vi "CM_DetectPulses.vi"(8 "Error In":errorcluster, 11 "Data":dbl[][](array[numeric])) -> (0 "Error out":errorcluster)   [LabVIEW 2016]
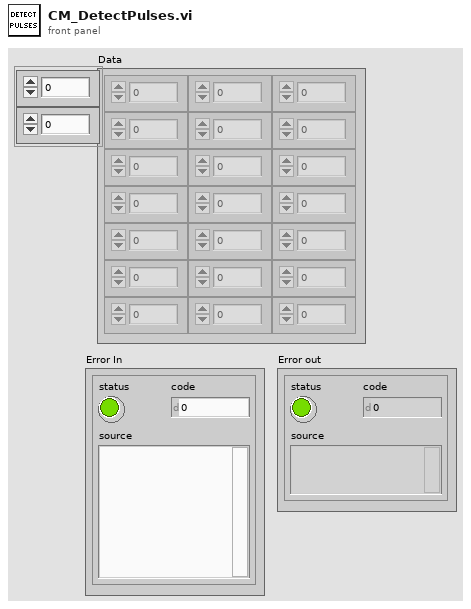
[diagram p1: front panel]
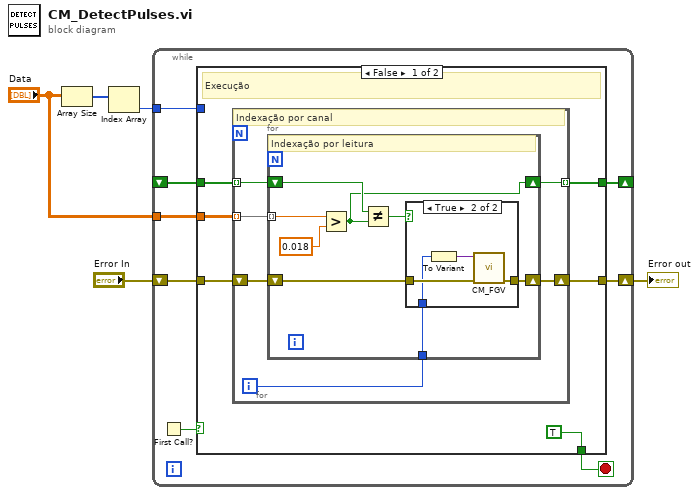
[diagram p0: block diagram]
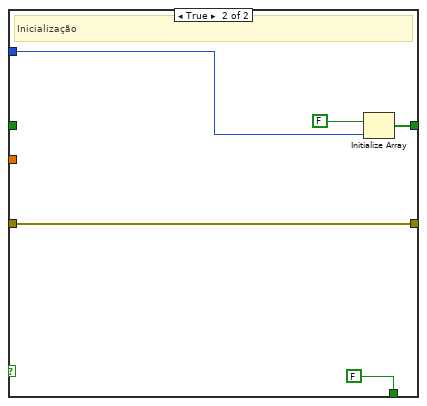
[diagram p3: hidden frame]
diagram:
  n1 = Array Size(array="Data") -> (size(s)=w5:i32[])
  n2 = Index Array(array=w5) -> (element=w4:i32)  [unwired: 1 in]
  n3 = while {
    tunnel: w4 -> [w12]
    shift-right: [w11] -> _
    shift-left: _ -> [w10]
    tunnel: "Data" -> [w9]
    shift-right: [w8] -> w1
    shift-left: "Error In" -> [w7]
    stop <- w13 stop-if-true
    n4 = First Call?() -> (First Call?: T/F=w6:bool)
    n5 = case shown="False" w6 {
      tunnel: [TRUE FALSE] -> w13
      tunnel: w12 -> [_ w42]
      tunnel: [w14 w40] -> w11
      tunnel: w10 -> [w18 _]
      tunnel: w9 -> [w17 _]
      tunnel: [w16 w39] -> w8
      tunnel: w7 -> [w15 w39]
      frame False {
        # "Execução"
        n6 = for {
          tunnel: w18 -> [w25] mode=indexing
          tunnel: w17 -> [w24] mode=indexing
          shift-right: [w23] -> w16
          shift-left: w15 -> [w22]
          tunnel: [w21] -> w14 mode=indexing
          i -> [w20]
          # "Indexação por canal"
          n7 = for {
            shift-right: [w30] -> w21
            shift-left: w25 -> [w31]
            tunnel: w24 -> [w33] mode=indexing
            shift-right: [w28] -> w23
            shift-left: w22 -> [w27]
            tunnel: w20 -> [w26]
            # "Indexação por leitura"
            n8 = Greater?(x=w33, y=0.018) -> (0:w30:bool)
            n9 = Not Equal?(x=w31, y=w30) -> (x != y?=w29:bool)
            n10 = case shown="True" w29 {
              tunnel: [w34 w38] -> w28
              tunnel: w27 -> [w34 w37]
              tunnel: w26 -> [_ w35]
              frame False {
              }
              frame True {
                n11 = To Variant(anything=w35) -> (Variant=w36:variant)
                n12 = call "CM_FGV.vi"("Error In"=w37, "DataIn"=w36) -> ("Error Out"=w38:errorcluster)  [unwired: 8 in, 1 out]
              }
            }
          }
        }
      }
      frame True {
        # "Inicialização"
        n13 = Initialize Array(FALSE, w42) -> (w40:bool[])
      }
    }
  }
  "Error out" <- w1
